vi "Facade.vi"(0 "Data In":T4={"low"=0, "high"=5}, 2 "Display State In":T2, 3 "Container State":T3) -> (6 "Data Out":T4={"low"=0, "high"=5}, 7 "Display State Out":T2, 8 "Action":T1)   [LabVIEW 2019, in "XVerticalSlide.xctl"]
uses:
  XVerticalSlide.xctl
  Data.ctl
  <vilib>/_xctls/Container State.ctl
  State.ctl
  <vilib>/_xctls/Action.ctl
  <vilib>/_xctls/XControlSupport.lvlib
panel:
  in  "Slide":cluster{i16, i16}(slide)={0, 5} scale=0.0..10.0
  # "1. Drop the controls that make up the appearance\nof the XControl here.\n\n2. Resize the window to fit the controls\n\n3. If the XControl is of fixed size,  make the \n window not resizable from VI Properties->Window Appearance.\n\n4. If you want the controls to automatically size when the XControl sizes, check  \"Scale all objects on front panel when window resizes\" in File->VI Properties->Window Size page.\n\n5. Show the block diagram and handle events for the controls on this panel."
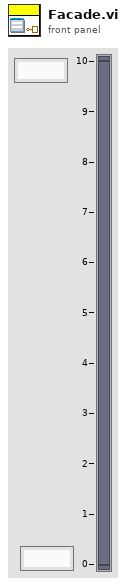
[diagram p1: front panel]
types:
  T1 = typedef "XControlSupport.lvlib/Action.ctl" = cluster{"Data Changed?":bool, "State Changed?":bool, "Action Name":string}
  T2 = typedef "XVerticalSlide.xctl/State.ctl" = cluster{"low":i16, "high":i16, "min":i16, "max":i16}
  T3 = typedef "XControlSupport.lvlib/Container State.ctl" = cluster{"Indicator?":bool, "Run Mode?":bool, " Refnum":refnum<vi>}
  T4 = typedef "XVerticalSlide.xctl/Data.ctl" = cluster{"low":i16, "high":i16}
  T5 = cluster{"[0]":i16, "[1]":i16, "[2]":i16, "[3]":i16, "[4]":i16, "[5]":i16, "[6]":i16, "[7]":i16, "[8]":i16}
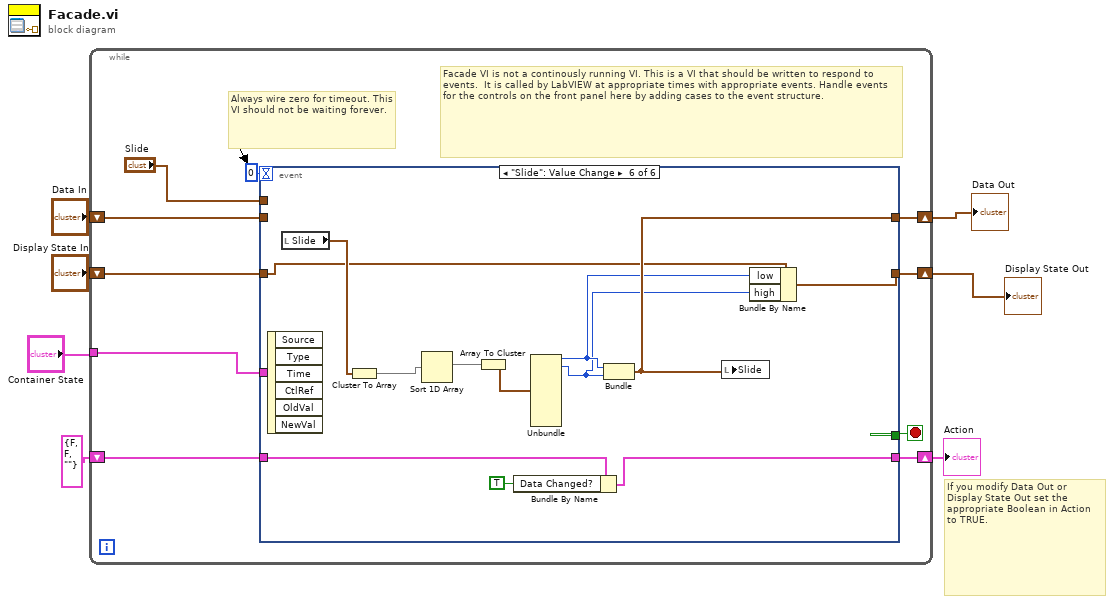
[diagram p0: block diagram]
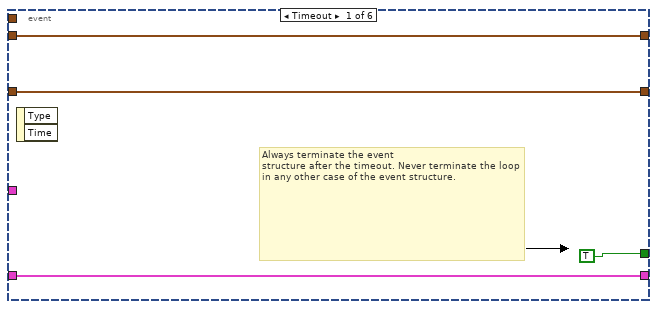
[diagram p2: hidden frame]
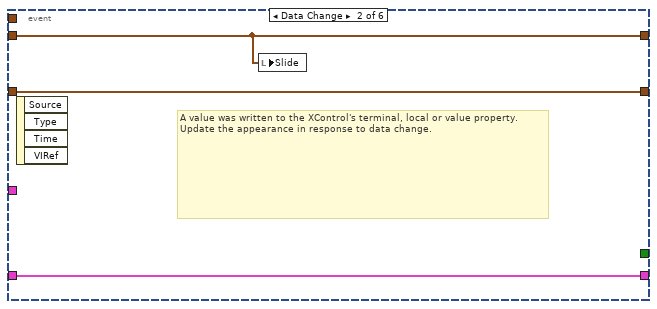
[diagram p3: hidden frame]
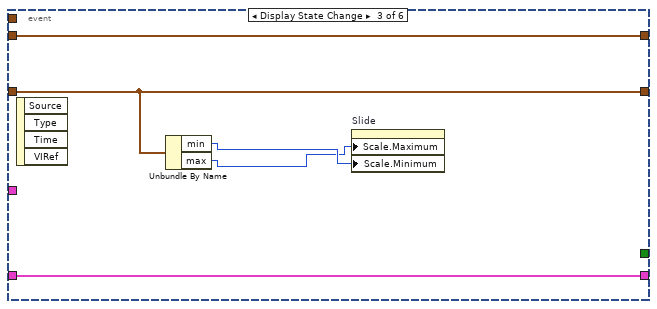
[diagram p4: hidden frame]
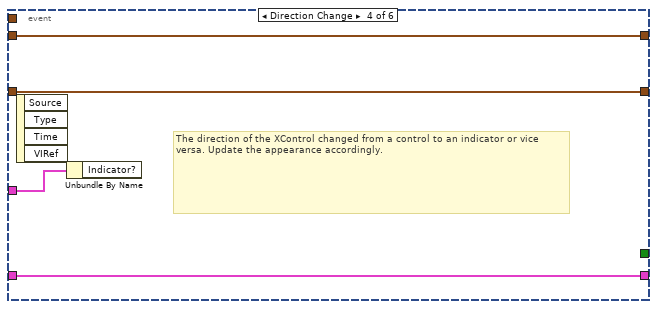
[diagram p5: hidden frame]
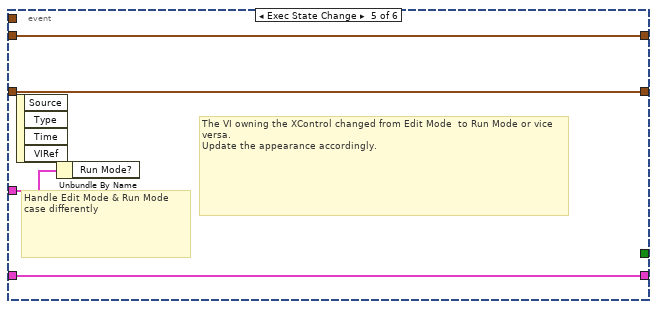
[diagram p6: hidden frame]
diagram:
  # "If you modify Data Out or\nDisplay State Out set the\nappropriate Boolean in Action\nto TRUE."
  n1 = while {
    shift-right: [w16] -> w4
    shift-left: "Display State In" -> [w17]
    tunnel: "Container State" -> [w13]
    shift-right: [w11] -> w7
    shift-left: "Data In" -> [w12]
    shift-right: [w9] -> w2
    shift-left: T1 {"Data Changed?"=FALSE, "State Changed?"=FALSE, "Action Name"=""} ("Action") -> [w10]
    stop <- w15 stop-if-true
    # "Facade VI is not a continously running VI. This is a VI that should be written to respond to events.  It is called by LabVIEW at appropriate times with appropriate events. Handle events for the controls on the front panel here by adding cases to the event structure."
    # "Always wire zero for timeout. This\nVI should not be waiting forever."
    n2 = event shown="[5] \"Slide\": Value Change" {
      selector: _ -> [_ _ _ _ _ _]
      dyn-events: _ -> [_ _ _ _ _ _]
      timeout: 0 -> [_ _ _ _ _ _]
      tunnel: w17 -> [w19 w24 w27 w32 w36 w40]
      tunnel: [w19 w24 w27 w32 w36 w41] -> w16
      tunnel: [TRUE _ _ _ _ _] -> w15
      tunnel: w13 -> [_ _ _ w33 w37 _]
      tunnel: w12 -> [w18 w22 w29 w31 w35 _]
      tunnel: [w18 w22 w29 w31 w35 w46] -> w11
      tunnel: [w20 w23 w28 w30 w34 w44] -> w9
      tunnel: w10 -> [w20 w23 w28 w30 w34 w45]
      tunnel: "Slide" -> [_ _ _ _ _ _]
      event Timeout {
        # "Always terminate the event\nstructure after the timeout. Never terminate the loop in any other case of the event structure."
        n3 = event-data() -> ()  [unwired: 1 in, 2 out]
      }
      event Data Change {
        # "A value was written to the XControl's terminal, local or value property.\nUpdate the appearance in response to data change."
        n4 = event-data() -> ()  [unwired: 1 in, 4 out]
        n5 = local write "Slide"(w22) -> ()
      }
      event Display State Change {
        n6 = event-data() -> ()  [unwired: 1 in, 4 out]
        n7 = Unbundle By Name(w27) -> ("min"=w26:i16, "max"=w25:i16)
        n8 = property on="Slide" class="Slide (strict)"("Scale.Maximum"=w25, "Scale.Minimum"=w26) -> ()  [unwired: 2 in, 2 out]
      }
      event Direction Change {
        # "The direction of the XControl changed from a control to an indicator or vice versa. Update the appearance accordingly."
        n9 = event-data() -> ()  [unwired: 1 in, 4 out]
        n10 = Unbundle By Name(w33) -> ()  [unwired: 1 out]
      }
      event Exec State Change {
        # "The VI owning the XControl changed from Edit Mode  to Run Mode or vice versa.\nUpdate the appearance accordingly."
        # "Handle Edit Mode & Run Mode\ncase differently"
        n11 = event-data() -> ()  [unwired: 1 in, 4 out]
        n12 = Unbundle By Name(w37) -> ()  [unwired: 1 out]
      }
      event "Slide": Value Change {
        n13 = event-data() -> ()  [unwired: 1 in, 6 out]
        n14 = local read "Slide"() -> (w42:cluster{i16, i16})
        n15 = Cluster To Array(cluster=w42) -> (array=w49:i16[])
        n16 = Sort 1D Array(array=w49) -> (sorted array=w48:i16[])
        n17 = Array To Cluster(array=w48) -> (cluster=w47:T5)
        n18 = Bundle By Name(cluster=w45, "Data Changed?"=TRUE) -> (w44:T1)
        n19 = Unbundle(w47) -> ("[0]"=w39:i16, "[1]"=w38:i16)  [unwired: 7 out]
        n20 = Bundle("[0]"=w39, "[1]"=w38) -> (w46:cluster{"[0]":i16, "[1]":i16})  [unwired: 1 in]
        n21 = local write "Slide"(w46) -> ()
        n22 = Bundle By Name(cluster=w40, "low"=w39, "high"=w38) -> (w41:T2)
      }
    }
  }
  "Display State Out" <- w4
  "Data Out" <- w7
  "Action" <- w2
